vi "Receive CCD Config.vi"(8 "error in (no error)":errorcluster, 11 "Stream in":refnum<class "Stream.lvclass">) -> (0 "error out":errorcluster, 3 "Stream out":refnum<class "Stream.lvclass">)   [LabVIEW 2018, in "Stream.lvclass"]
uses:
  Stream.lvclass
  Interface/Interface.lvclass
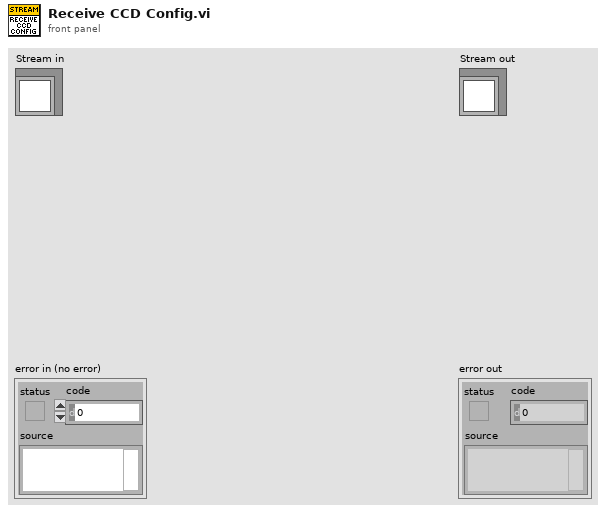
[diagram p1: front panel]
types:
  T1 = cluster{"Exposure Time":dbl, "Pre-amp gain":u8, "Readout Rate":u8, "EM Mode":u8, "EM Gain":u16, "Binning":u16, "Initial Line":u16, "Initial Cloumn":u16, "Final Line":u16, "Final Column":u16, "Kinetic Series Length":u32, "Shutter Mode":u8, "Cooler ON/OFF":u16, "Temperature":i8, "Image Name":string, "Image Path":string}
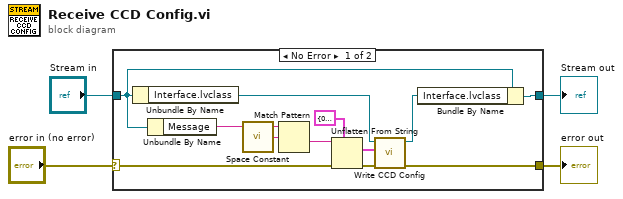
[diagram p0: block diagram]
diagram:
  n1 = case shown="No Error" "error in (no error)" {
    selector: "error in (no error)" -> [w16 w18]
    tunnel: [w10 w18] -> w3
    tunnel: [w12 w17] -> w1
    tunnel: "Stream in" -> [w11 w17]
    frame No Error {
      n2 = Unbundle By Name(w11) -> ("Interface.lvclass"=w7:refnum<class "Interface.lvclass">)
      n3 = Unbundle By Name(w11) -> ("Message"=w14:string)
      n4 = call <vilib>:"Space Constant.vi"() -> ("String"=w15:string)
      n5 = Match Pattern(string=w14, regular expression=w15) -> (after substring=w13:string)  [unwired: 1 in, 3 out]
      n6 = Unflatten From String(type=T1 {"Exposure Time"=0.1, "Pre-amp gain"=0, "Readout Rate"=0, "EM Mode"=0, "EM Gain"=2, "Binning"=1, "Initial Line"=1, "Initial Cloumn"=1, "Final Line"=1024, "Final Column"=1024, "Kinetic Series Length"=1, "Shutter Mode"=2, "Cooler ON/OFF"=0, "Temperature"=20, "Image Name"="", "Image Path"=""} ("CCD Config"), binary string=w13, error in (no error)=w16) -> (value=w8:T1, error out=w9:errorcluster)  [unwired: 2 in, 1 out]
      n7 = call "Write CCD Config.vi"("error in (no error)"=w9, "CCD Config"=w8, "Interface in"=w7) -> ("error out"=w10:errorcluster, "Interface out"=w6:refnum<class "Interface.lvclass">)  [unwired: 7 in]
      n8 = Bundle By Name(cluster=w11, "Interface.lvclass"=w6) -> (w12:refnum<class "Stream.lvclass">)
    }
    frame Error {
    }
  }
  "error out" <- w3
  "Stream out" <- w1
